vi "Raw Data Interpretor.vi"(1 "Sensor Data":dbl[][](array[numeric]) format="%0.2f") -> (0 "Interpreted Data":dbl[][](array[numeric]) format="%0.2f")   [LabVIEW 2013]
doc: "Interpret raw sensor data by applying transformations and calibrations to it."
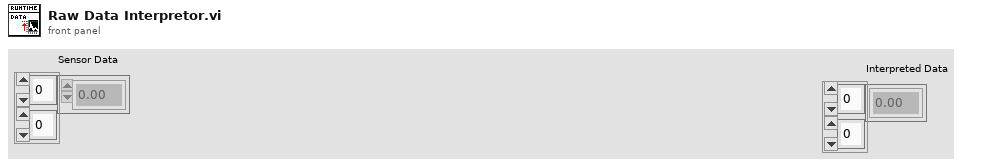
[diagram p1: front panel]
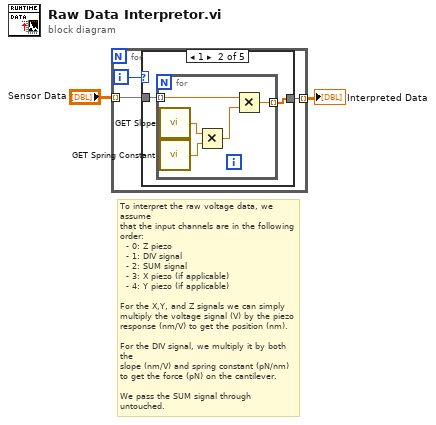
[diagram p0: block diagram]
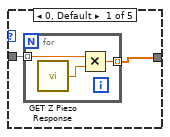
[diagram p2: hidden frame]
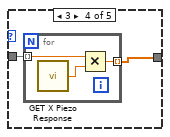
[diagram p4: hidden frame]
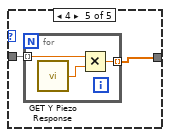
[diagram p5: hidden frame]
diagram:
  # "To interpret the raw voltage data, we assume\nthat the input channels are in the following\norder:\n  - 0: Z piezo\n  - 1: DIV signal\n  - 2: SUM signal\n  - 3: X piezo (if applicable)\n  - 4: Y piezo (if applicable)\n\nFor the X,Y, and Z signals we can simply \nmultiply the voltage signal (V) by the piezo\nresponse (nm/V) to get the position (nm).\n\nFor the DIV signal, we multiply it by both the\nslope (nm/V) and spring constant (pN/nm)\nto get the force (pN) on the cantilever.\n\nWe pass the SUM signal through untouched."
  n1 = for {
    tunnel: "Sensor Data" -> [w3] mode=indexing
    tunnel: [w4] -> w1 mode=indexing
    i -> [w5]
    n2 = case shown="1" w5 {
      tunnel: [w6 w11 w18 w19 w24] -> w4
      tunnel: w3 -> [w7 w12 w18 w20 w25]
      frame 0, Default {
        n3 = for {
          tunnel: w7 -> [w10] mode=indexing
          tunnel: [w8] -> w6 mode=indexing
          n4 = call "GET Z Piezo Response.vi"() -> ("Z Piezo Response"=w9:dbl)
          n5 = Multiply(x=w10, y=w9) -> (x*y=w8:dbl)
        }
      }
      frame 1 {
        n6 = for {
          tunnel: w12 -> [w17] mode=indexing
          tunnel: [w16] -> w11 mode=indexing
          n7 = call "GET Slope.vi"() -> ("Slope"=w14:dbl)
          n8 = call "GET Spring Constant.vi"() -> ("Spring Constant"=w13:dbl)
          n9 = Multiply(x=w14, y=w13) -> (x*y=w15:dbl)
          n10 = Multiply(x=w17, y=w15) -> (x*y=w16:dbl)
        }
      }
      frame 2 {
      }
      frame 3 {
        n11 = for {
          tunnel: w20 -> [w23] mode=indexing
          tunnel: [w21] -> w19 mode=indexing
          n12 = call "GET X Piezo Response.vi"() -> ("X Piezo Response"=w22:dbl)
          n13 = Multiply(x=w23, y=w22) -> (x*y=w21:dbl)
        }
      }
      frame 4 {
        n14 = for {
          tunnel: w25 -> [w28] mode=indexing
          tunnel: [w26] -> w24 mode=indexing
          n15 = call "GET Y Piezo Response.vi"() -> ("Y Piezo Response"=w27:dbl)
          n16 = Multiply(x=w28, y=w27) -> (x*y=w26:dbl)
        }
      }
    }
  }
  "Interpreted Data" <- w1
